vi "FRCts20_Backend_Test_TeamRoot_POST.vi"(8 "error in (no error)":errorcluster, 11 "TeamRoot In":T1={"Teams"=[{"Team Index"=0, "Team Number"=54321, "Team ID"=0, "Team Name"="a", "Short Team Name"="b", "Nick Name"="c", "Robot Name"="d", "City"="e", "State"="f", "Country"="g", "Rookie Year"=1989, "SWType"="unknown", "CAN"=TRUE, "Vision"=TRUE, "Kinect"=TRUE, "Tags"="h", "Avatar"="i", "Events"=[]}], "APIReturn"=""}) -> (0 "error out":errorcluster, 1 "Time (ms)":u32, 2 "Status":string, 3 "Team Root":T1, 5 "Success":bool)   [LabVIEW 2014, in "FRCts20_Backend_TestCode.lvlib"]
uses:
  FRCts20_Backend_TestCode.lvlib
  FRCts20_Backend_API/FRCts20_Backend_API_TeamRoot.ctl
  FRCts20_Backend_API/FRCts20_Backend_API_SW.ctl
  FRCts20_Backend_API/FRCts20_Backend_API_Command_TeamRoot.ctl
  FRCts20_Backend_API/FRCts20_Backend_API_TeamRoot.vi
  FRCts20_Backend_API/FRCts20_Backend_API.lvlib
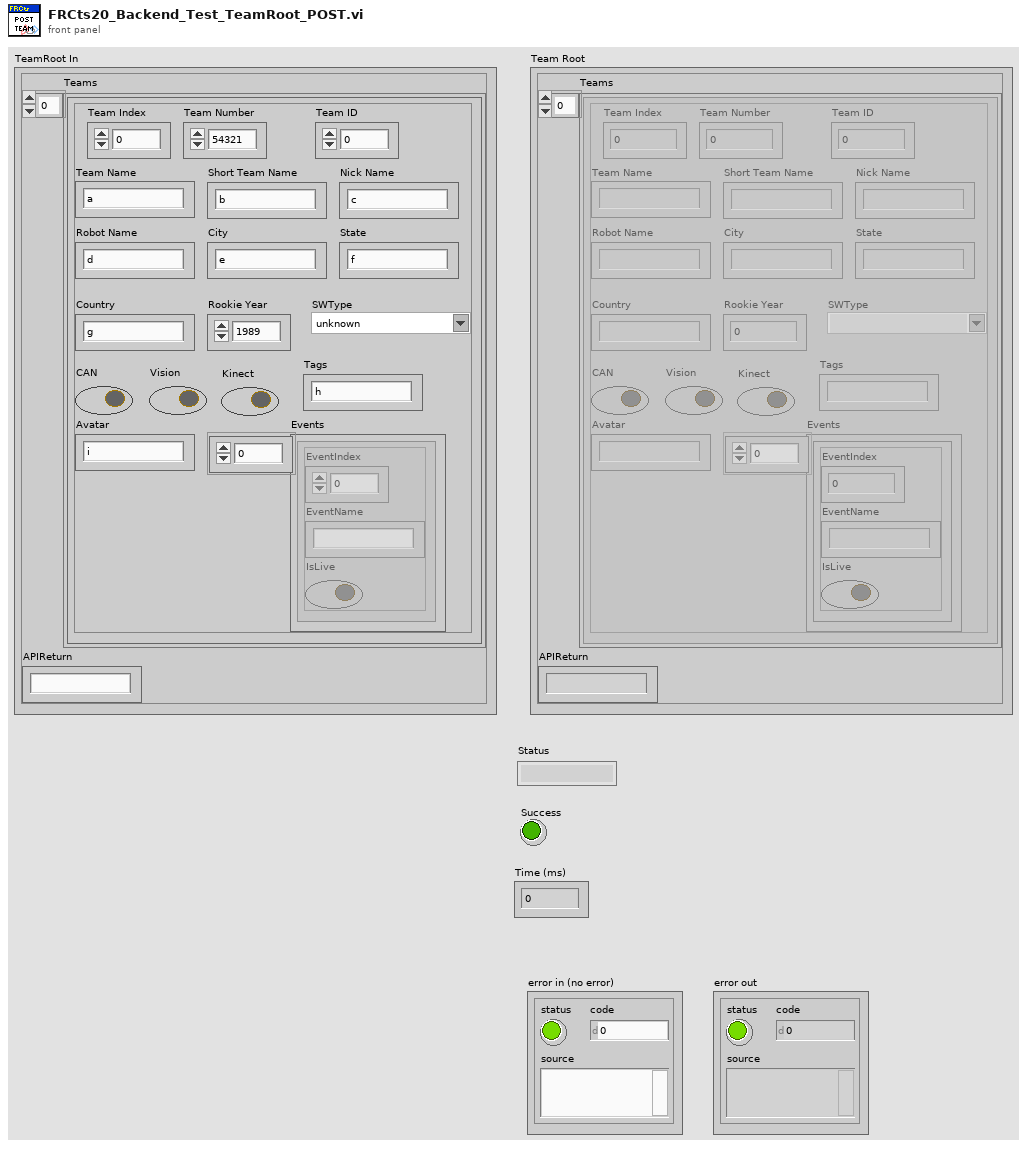
[diagram p1: front panel]
types:
  T1 = typedef "FRCts20_Backend_API.lvlib/FRCts20_Backend_API_TeamRoot.ctl" = cluster{"Teams":cluster{"Team Index":u32, "Team Number":u32, "Team ID":u32, "Team Name":string, "Short Team Name":string, "Nick Name":string, "Robot Name":string, "City":string, "State":string, "Country":string, "Rookie Year":u32, "SWType":T2, "CAN":bool, "Vision":bool, "Kinect":bool, "Tags":string, "Avatar":string, "Events":cluster{"EventIndex":u32, "EventName":string, "IsLive":bool}[]}[], "APIReturn":string}
  T2 = typedef "FRCts20_Backend_API.lvlib/FRCts20_Backend_API_SW.ctl" = string
  T3 = typedef "FRCts20_Backend_API.lvlib/FRCts20_Backend_API_Command_TeamRoot.ctl" = string
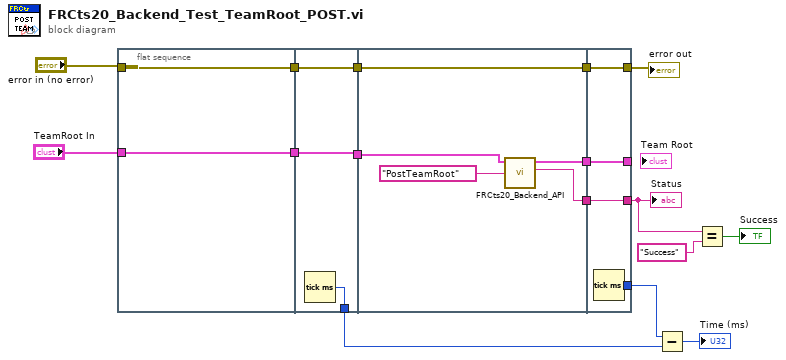
[diagram p0: block diagram]
diagram:
  n1 = flat-sequence {
    tunnel: "error in (no error)" -> [w18]
    tunnel: [w18] -> w16
    tunnel: [w17] -> w3
    tunnel: "TeamRoot In" -> [w17]
    tunnel: [w21] -> w5
    tunnel: [w20] -> w15
    tunnel: w16 -> [w20]
    tunnel: w3 -> [w19]
    tunnel: [w19] -> w1
    tunnel: [w26] -> w14
    tunnel: w15 -> [w26]
    tunnel: [w25] -> w13
    tunnel: [w24] -> w12
    tunnel: w1 -> [w22]
    tunnel: [w30] -> w6
    tunnel: [w29] -> w8
    tunnel: w14 -> [w29]
    tunnel: [w28] -> _
    tunnel: w13 -> [w28]
    tunnel: [w27] -> w4
    tunnel: w12 -> [w27]
    frame #0 {
    }
    frame #1 {
      n2 = Tick Count (ms)() -> (millisecond timer value=w21:u32)
    }
    frame #2 {
      n3 = call-poly "FRCts20_Backend_API.vi"("Command"=T3 "PostTeamRoot", "Team In"=w22) -> ("Status"=w24:string, "Team Out"=w25:T1)  [unwired: 7 in, 1 out]
    }
    frame #3 {
      n4 = Tick Count (ms)() -> (millisecond timer value=w30:u32)
    }
  }
  n5 = Subtract(x=w6, y=w5) -> (x-y=→"Time (ms)":u32)
  n6 = Equal?(x=w4, y="Success") -> (x = y?=→"Success":bool)
  "Status" <- w4
  "error out" <- w8
